vi "Shutdown Module.vi"(7 "Coordinate Space":refnum<k21>="Coordinate Space 1", 8 "error in (no error)":errorcluster, 11 "Axis Resources In":refnum<k21>[](array[refnum])) -> (0 "error out":errorcluster, 3 "Axis Resources Out":refnum<k21>[](array[refnum]))   [LabVIEW 2014]
uses:
  <vilib>/Motion/Express/_s/nimc.ex.stopMove.stop.coordinate.modeDecelerate.vi
  <vilib>/Motion/Express/_s/nimc.ex.power.power.axis.vi
  <vilib>/Motion/BlockNode/FB.NIMotion.xnode
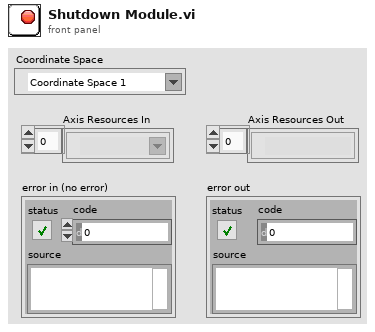
[diagram p1: front panel]
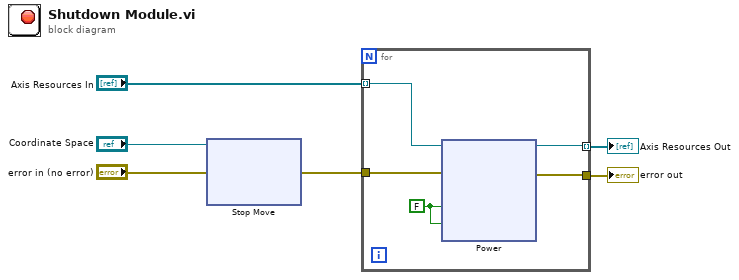
[diagram p0: block diagram]
diagram:
  n1 = xnode ("Stop Move")("resource"="Coordinate Space", "error in"="error in (no error)") -> ("error out"=w2:errorcluster)  [unwired: 1 in, 2 out]
  n2 = for {
    tunnel: "Axis Resources In" -> [w8] mode=indexing
    tunnel: w2 -> [w7]
    tunnel: [w10] -> w6
    tunnel: [w9] -> w5 mode=indexing
    w11 = FALSE ("enable axis")
    n3 = xnode ("Power")("enable axis"=w11, "enable drive"=w11, "resource"=w8, "error in"=w7) -> ("resource out"=w9:refnum<k21>, "error out"=w10:errorcluster)
  }
  "error out" <- w6
  "Axis Resources Out" <- w5
